vi "Model - Get Elevator States.vi"(8 "error in (no error)":errorcluster, 11 "View Model":T2) -> (0 "error out":errorcluster, 1 "Next Elevator State":T1, 2 "Elevator State":T1, 3 "View Model":T2)   [LabVIEW 2013]
doc: "Returns the current and next elevator states."
uses:
  Controls/View Model.ctl
  Error/Controls/Error Model.ctl
  Error/Controls/Error Types.ctl
  Controls/Shared Model.ctl
  Elevator Controller/Controls/Elevator Model.ctl
  Elevator Controller/Controls/Controller Overhead.ctl
  Elevator Controller/Controls/Elevator States.ctl
  Elevator Controller/Controls/Elevator Location.ctl
  Elevator Controller/Controls/Elevator Command Event.ctl
  Elevator Controller/Controls/Elevator Commands.ctl
  Configuration/Controls/Configuration Model.ctl
  Configuration/Controls/Configuration Data.ctl
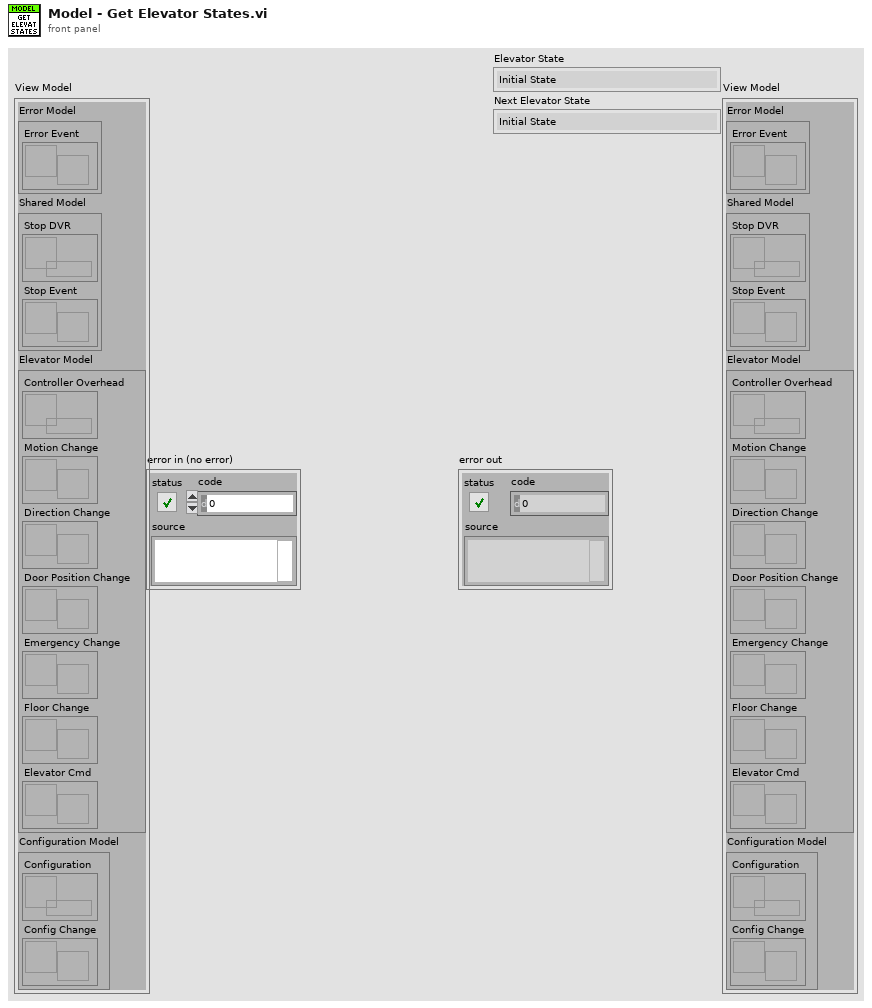
[diagram p1: front panel]
types:
  T1 = typedef "Elevator States.ctl" = enum16{"Initial State", "Open Doors", "Close Doors", "Start Move", "Move", "Finish Move", "Emergency", "Analysis"}
  T2 = typedef "View Model.ctl" = cluster{"Error Model":T3, "Shared Model":T4, "Elevator Model":T5, "Configuration Model":T6}
  T3 = typedef "Error Model.ctl" = cluster{"Error Event":refnum<user-event>}
  T4 = typedef "Shared Model.ctl" = cluster{"Stop DVR":refnum<data-value>, "Stop Event":refnum<user-event>}
  T5 = typedef "Elevator Model.ctl" = cluster{"Controller Overhead":refnum<data-value>, "Motion Change":refnum<user-event>, "Direction Change":refnum<user-event>, "Door Position Change":refnum<user-event>, "Emergency Change":refnum<user-event>, "Floor Change":refnum<user-event>, "Elevator Cmd":refnum<user-event>}
  T6 = typedef "Configuration Model.ctl" = cluster{"Configuration":refnum<data-value>, "Config Change":refnum<user-event>}
  T7 = typedef "Controller Overhead.ctl" = cluster{"In Motion?":bool, "Direction":bool, "Door Movement":bool, "Elevator State":T1, "Next Elevator State":T1, "Timer":dbl, "Elapsed Time":dbl, "Door Position":bool}
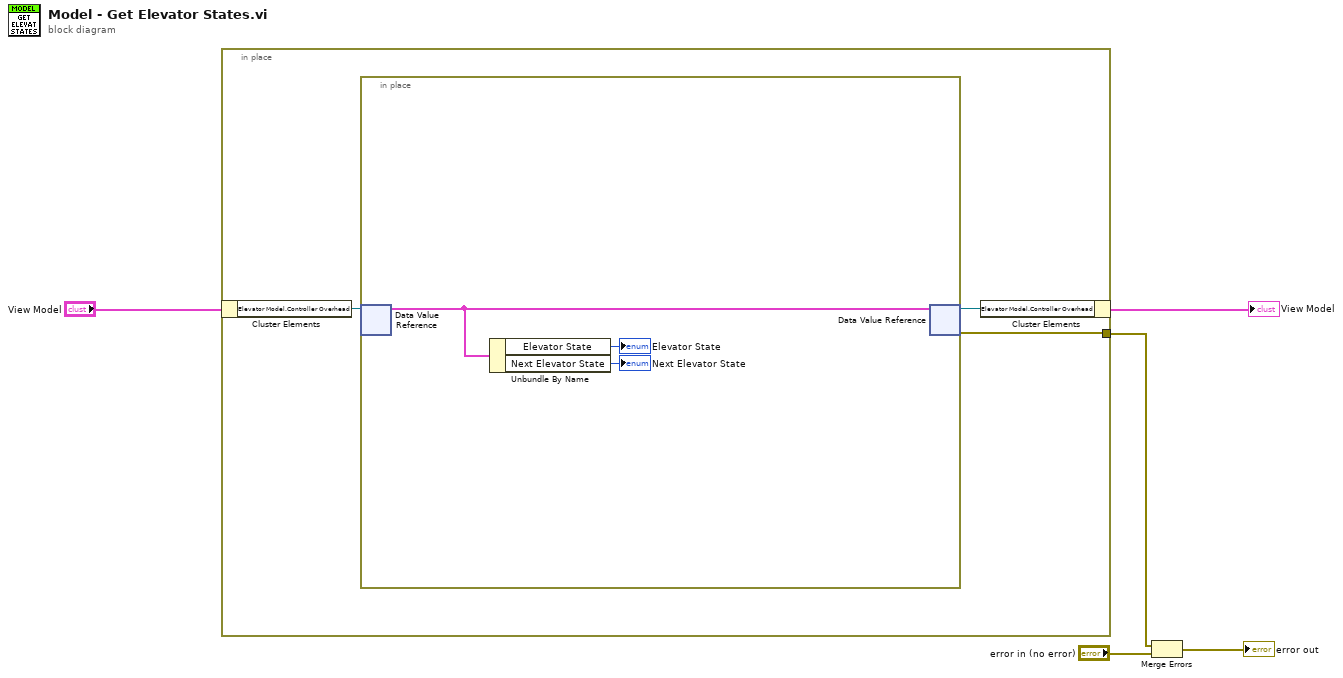
[diagram p0: block diagram]
diagram:
  n1 = in-place {
    in-place-border: [w6] -> w4
    n2 = in-place-cluster #1("View Model") -> ("Elevator Model.Controller Overhead"=w8:refnum<data-value>)
    n3 = in-place {
      n4 = in-place-dvr #2(w8) -> (w11:T7)  [unwired: 1 out]
      n5 = Unbundle By Name(w11) -> ("Elevator State"=→"Elevator State":T1, "Next Elevator State"=→"Next Elevator State":T1)
      n6 = in-place-dvr #2(w11) -> (w7:refnum<data-value>, w6:errorcluster)
    }
    n7 = in-place-cluster #1("Elevator Model.Controller Overhead"=w7) -> (→"View Model":T2)
  }
  n8 = Merge Errors(w4, "error in (no error)") -> (→"error out":errorcluster)
